vi "Format Technique (Depreciated).vi"(8 "error in (no error)":errorcluster, 9 "Technique in":T1, 10 "Technique Parameters in":variant, 11 "Potentiostat Galvanostat in":refnum<class "Potentiostat Galvanostat.lvclass">) -> (0 "error out":errorcluster, 1 "Technique Parameters out":T2 {"Parameter Type" items=["I32 (Long)", "BOOL (Boolean)", "SGL (Single Precision)"]}, 3 "Potentiostat Galvanostat out":refnum<class "Potentiostat Galvanostat.lvclass">)   [LabVIEW 2018, in "Potentiostat Galvanostat.lvclass"]
uses:
  Potentiostat Galvanostat.lvclass
  Controls/Technique Parameters.ctl
  Controls/Technique Parameter.ctl
  Controls/Parameter Type.ctl
  Controls/Technique List.ctl
  Controls/CA Parameters.ctl
  Controls/CA Internal Parameters.ctl
  Controls/CP Internal Parameters.ctl
  Controls/CP Parameters.ctl
  Controls/OCV Internal Parameters.ctl
  Controls/OCV Parameters.ctl
  Controls/CV Internal Parameters.ctl
  Controls/CV Parameters.ctl
  Controls/PEIS Internal Parameters.ctl
  Controls/PEIS Parameters.ctl
  Controls/GEIS Internal Parameters.ctl
  Controls/GEIS Parameters.ctl
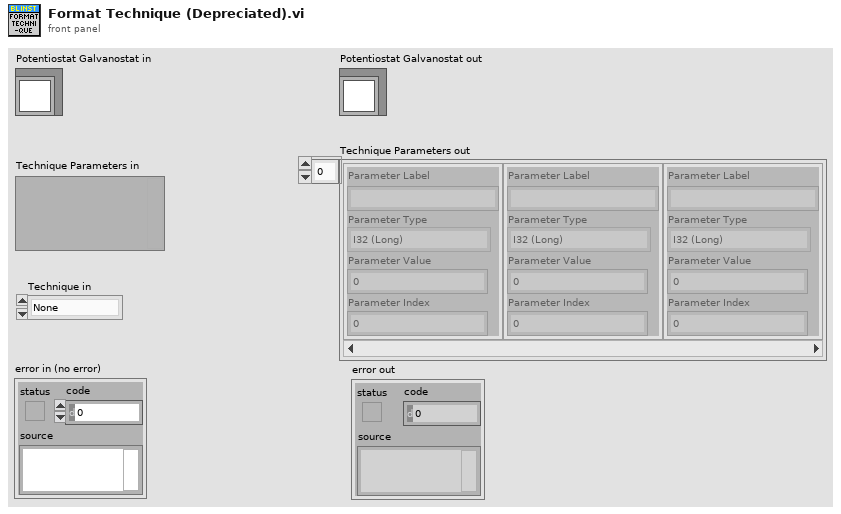
[diagram p1: front panel]
types:
  T1 = typedef "Potentiostat Galvanostat.lvclass/Technique List.ctl" = enum16{"None", "ocv", "cv", "biovscan", "ca", "cp", "iscan", "vscan", "lasv", "load", "pow", "peis", "geis", "seisp", "seisg", "dpv", "swv", "npv", "mpv", "dnpv", "dpa", "evt", "lp", "gc", "cpp", "pdp", "psp", "zra", "ircmp", "pzir", "gzir", "loop", "TO", "TI", "TOS", "vscanlimit", "iscanlimit", "mp", "casp", "casg", "calimit", "cplimit"}
  T2 = typedef "Potentiostat Galvanostat.lvclass/Technique Parameters.ctl" = T3[]
  T3 = typedef "Potentiostat Galvanostat.lvclass/Technique Parameter.ctl" = cluster{"Parameter Label":string, "Parameter Type":T4, "Parameter Value":i32, "Parameter Index":i32}
  T4 = typedef "Potentiostat Galvanostat.lvclass/Parameter Type.ctl" = i32
  T5 = typedef "Potentiostat Galvanostat.lvclass/GEIS Parameters.ctl" = cluster{"Initial frequency (Hz)":sgl, "sweep linear/logarithmic":bool, "Number of frequencies":i32, "Final frequency (Hz)":sgl, "Sine amplitude (A)":sgl, "No. of repeat times":i32, "No. of period to wait\nbefore each frequency":sgl, "Non-stationary correction":bool, "I Range":u16, "Bandwidth":u16, "CE to ground Mode":u16, "Step duration (s)":sgl, "Record every dE (V)":sgl, "Record every dt (s)":sgl, "Initial current step (A)":sgl, "Current step vs initial one":bool}
  T6 = typedef "Potentiostat Galvanostat.lvclass/GEIS Internal Parameters.ctl" = cluster{"Step_number":i32, "Initial_Current_step":sgl, "vs_initial ":bool, "Final_Current_step":sgl, "vs_final":bool, "Duration_step":sgl, "Record_every_dE":sgl, "Record_every_dT":sgl, "Initial_frequency":sgl, "sweep":bool, "Final_frequency":sgl, "Frequency_number":i32, "Amplitude_Current":sgl, "Wait_for_steady":sgl, "Average_N_times":i32, "Correction":bool, "I_Range":u16, "Bandwidth":u16, "em":u16, "ce":u16}
  T7 = typedef "Potentiostat Galvanostat.lvclass/PEIS Parameters.ctl" = cluster{"Step duration (s)":sgl, "Record every dI (A)":sgl, "Record every dt (s)":sgl, "Initial voltage step (V)":sgl, "Voltage step vs initial one":bool, "Initial frequency (Hz)":sgl, "sweep linear/logarithmic":bool, "Number of frequencies":i32, "Final frequency (Hz)":sgl, "Sine amplitude (V)":sgl, "No. of repeat times":i32, "No. of period to wait\nbefore each frequency":sgl, "Non-stationary correction":bool, "I Range":u16, "Bandwidth":u16, "CE to ground Mode":u16}
  T8 = typedef "Potentiostat Galvanostat.lvclass/PEIS Internal Parameters.ctl" = cluster{"Step_number":i32, "Initial_Voltage_step":sgl, "vs_initial":bool, "Final_Voltage_step":sgl, "vs_final":bool, "Duration_step":sgl, "Record_every_dI":sgl, "Record_every_dT":sgl, "Initial_frequency":sgl, "sweep":bool, "Final_frequency":sgl, "Frequency_number":i32, "Amplitude_Voltage":sgl, "Wait_for_steady":sgl, "Average_N_times":i32, "Correction":bool, "I_Range":u16, "Bandwidth":u16, "em":u16, "ce":u16}
  T9 = typedef "Potentiostat Galvanostat.lvclass/CV Parameters.ctl" = cluster{"Ei Params":cluster{"Current step vs initial one (Ei)":bool, "Voltage step (V) (Ei)":sgl, "slew rate array (mV/s) (Ei)":sgl}, "E1 Params":cluster{"Current step vs initial one (E1)":bool, "Voltage step (V) (E1)":sgl, "slew rate array (mV/s) (E1)":sgl}, "E2 Params":cluster{"Current step vs initial one (E2)":bool, "Voltage step (V) (E2)":sgl, "slew rate array (mV/s) (E2)":sgl}, "Ef Params":cluster{"Current step vs initial one (Ef)":bool, "Voltage step (V) (Ef)":sgl, "slew rate array (mV/s) (Ef)":sgl}, "Number of cycle":i32, "recording on dE (V)":sgl, "average every dE":bool, "Begin step accumulation (1 = 100% of step)":sgl, "End step accumulation ( 1 = 100% of step)":sgl, "I range":u16, "Bandwidth":u16, "Ewe range":u16, "CE to ground Mode":u16}
  T10 = typedef "Potentiostat Galvanostat.lvclass/CV Internal Parameters.ctl" = cluster{"Voltage_steps":cluster{"vs_initial":bool, "Voltage_step":sgl, "Scan_Rate":sgl}[], "N_Cycles":i32, "Record_every_dE":sgl, "Average_over_dE":bool, "Begin_measuring_I":sgl, "End_measuring_I":sgl, "I_Range":u16, "E_Range":u16, "Bandwidth":u16, "em":u16, "ce":u16, "Scan_number":u16, "tb":sgl}
  T11 = typedef "Potentiostat Galvanostat.lvclass/OCV Parameters.ctl" = cluster{"Rest duration (s)":sgl, "Record every dE (V)":sgl, "Record every dT (s)":sgl, "Ewe range":u16, "CE to ground Mode":u16}
  T12 = typedef "Potentiostat Galvanostat.lvclass/OCV Internal Parameters.ctl" = cluster{"Rest_time_T":sgl, "Record_every_dE":sgl, "Record_every_dT":sgl, "E_Range":u16, "em":u16, "ce":u16, "tb":sgl}
  T13 = typedef "Potentiostat Galvanostat.lvclass/CP Parameters.ctl" = cluster{"Current Steps":cluster{"Current step vs initial\none":bool, "Current step (A)":sgl, "Duration step (s)":sgl}[], "No. of steps":i32, "Record every dt (s)":sgl, "Record every dE (V)":sgl, "No. of times\ntechnique is repeated":i32, "I range":u16, "Ewe range":u16, "Bandwidth":u16, "CE to ground Mode":u16}
  T14 = typedef "Potentiostat Galvanostat.lvclass/CP Internal Parameters.ctl" = cluster{"Current_steps":cluster{"vs_initial":bool, "Current_step":sgl, "Duration_step":sgl}[], "Step_number":i32, "N_Cycles":i32, "Record_every_dE":sgl, "Record_every_dT":sgl, "I_Range":u16, "E_Range":u16, "Bandwidth":u16, "em":u16, "ce":u16, "tb":sgl}
  T15 = typedef "Potentiostat Galvanostat.lvclass/CA Internal Parameters.ctl" = cluster{"tb":sgl, "Voltage_steps":cluster{"vs_initial":bool, "Voltage_step":sgl, "Duration_step":sgl}[], "Step_number":i32, "N_Cycles":i32, "Record_every_dI":sgl, "Record_every_dT":sgl, "I_Range":u16, "E_Range":u16, "Bandwidth":u16, "em":u16, "ce":u16}
  T16 = typedef "Potentiostat Galvanostat.lvclass/CA Parameters.ctl" = cluster{"Voltage Steps":cluster{"Voltage step vs initial one":bool, "Voltage step (V)":sgl, "Duration step (s)":sgl}[], "No. of steps":i32, "Record every dt (s)":sgl, "Record every dI (A)":sgl, "No. of times\ntechnique is repeated":i32, "I range":u16, "Ewe range":u16, "Bandwidth":u16, "CE to ground Mode":u16}
  T17 = cluster{"Voltage step vs initial one":bool, "Voltage step (V)":sgl, "Duration step (s)":sgl}[]
  T18 = cluster{"Current step vs initial\none":bool, "Current step (A)":sgl, "Duration step (s)":sgl}[]
  T19 = cluster{"Current step vs initial one (Ei)":bool, "Voltage step (V) (Ei)":sgl, "slew rate array (mV/s) (Ei)":sgl}
  T20 = cluster{"Current step vs initial one (E1)":bool, "Voltage step (V) (E1)":sgl, "slew rate array (mV/s) (E1)":sgl}
  T21 = cluster{"Current step vs initial one (E2)":bool, "Voltage step (V) (E2)":sgl, "slew rate array (mV/s) (E2)":sgl}
  T22 = cluster{"Current step vs initial one (Ef)":bool, "Voltage step (V) (Ef)":sgl, "slew rate array (mV/s) (Ef)":sgl}
  T23 = cluster{"Current step vs initial one (Ef)":bool, "Voltage step (V) (Ef)":sgl, "slew rate array (mV/s) (Ef)":sgl}[]
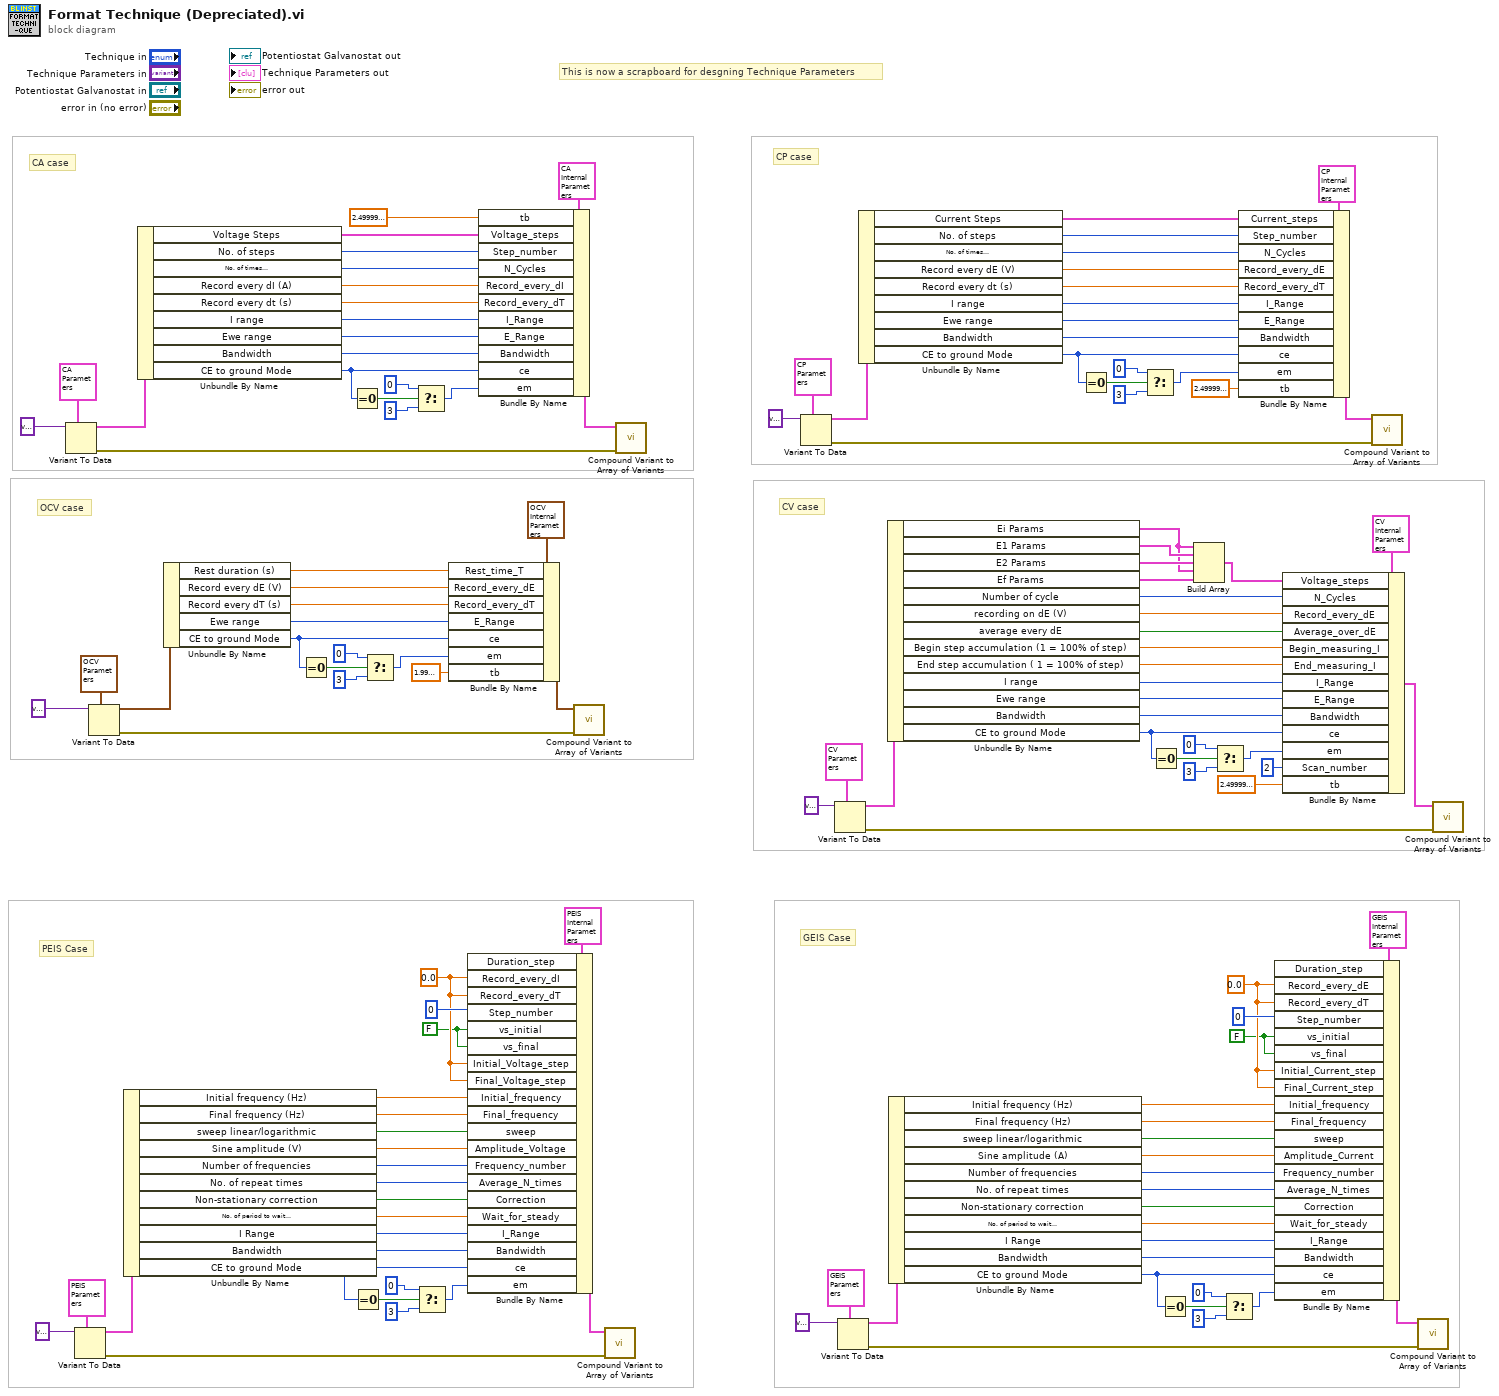
[diagram p0: block diagram]
diagram:
  w18 = FALSE ("vs_initial")
  w19 = sgl 0.0 ("Duration_step")
  w26 = FALSE ("vs_initial")
  w27 = sgl 0.0 ("Duration_step")
  # "This is now a scrapboard for desgning Technique Parameters"
  # "GEIS Case"
  # "PEIS Case"
  # "CV case"
  # "OCV case"
  # "CP case"
  # "CA case"
  n1 = Variant To Data(type=T16 {"Voltage Steps"=[{"Voltage step vs initial one"=TRUE, "Voltage step (V)"=0.0, "Duration step (s)"=1.0}, {"Voltage step vs initial one"=TRUE, "Voltage step (V)"=0.1, "Duration step (s)"=1.0}, {"Voltage step vs initial one"=TRUE, "Voltage step (V)"=0.2, "Duration step (s)"=1.0}], "No. of steps"=2, "Record every dt (s)"=0.01, "Record every dI (A)"=1e-05, "No. of times\ntechnique is repeated"=0, "I range"=12, "Ewe range"=3, "Bandwidth"=5, "CE to ground Mode"=0} ("CA Parameters"), Variant=variant ("Technique Parameters in")) -> (data=w114:T16, error out=w111:errorcluster)  [unwired: 1 in]
  n2 = Variant To Data(type=T7 {"Step duration (s)"=1.0, "Record every dI (A)"=0.1, "Record every dt (s)"=0.1, "Initial voltage step (V)"=0.0, "Voltage step vs initial one"=TRUE, "Initial frequency (Hz)"=0.0, "sweep linear/logarithmic"=TRUE, "Number of frequencies"=51, "Final frequency (Hz)"=1.0, "Sine amplitude (V)"=0.01, "No. of repeat times"=1, "No. of period to wait\nbefore each frequency"=2.0, "Non-stationary correction"=TRUE, "I Range"=12, "Bandwidth"=5, "CE to ground Mode"=0} ("PEIS Parameters"), Variant=variant ("Technique Parameters in")) -> (data=w25:T7, error out=w30:errorcluster)  [unwired: 1 in]
  n3 = Variant To Data(type=T11 {"Rest duration (s)"=1.0, "Record every dE (V)"=0.01, "Record every dT (s)"=0.01, "Ewe range"=3, "CE to ground Mode"=0} ("OCV Parameters"), Variant=variant ("Technique Parameters in")) -> (data=w79:T11, error out=w76:errorcluster)  [unwired: 1 in]
  n4 = Unbundle By Name(w25) -> ("Initial frequency (Hz)"=w48:sgl, "Final frequency (Hz)"=w47:sgl, "sweep linear/logarithmic"=w46:bool, "Sine amplitude (V)"=w45:sgl, "Number of frequencies"=w44:i32, "No. of repeat times"=w43:i32, "Non-stationary correction"=w42:bool, "No. of period to wait\nbefore each frequency"=w41:sgl, "I Range"=w40:u16, "Bandwidth"=w39:u16, "CE to ground Mode"=w33:u16)
  n5 = Unbundle By Name(w114) -> ("Voltage Steps"=w127:T17, "No. of steps"=w128:i32, "No. of times\ntechnique is repeated"=w126:i32, "Record every dI (A)"=w125:sgl, "Record every dt (s)"=w124:sgl, "I range"=w121:u16, "Ewe range"=w122:u16, "Bandwidth"=w123:u16, "CE to ground Mode"=w116:u16)
  n6 = Unbundle By Name(w79) -> ("Rest duration (s)"=w89:sgl, "Record every dE (V)"=w88:sgl, "Record every dT (s)"=w87:sgl, "Ewe range"=w86:u16, "CE to ground Mode"=w81:u16)
  n7 = Equal To 0?(x=w81) -> (x = 0?=w84:bool)
  n8 = Equal To 0?(x=w116) -> (x = 0?=w119:bool)
  n9 = Equal To 0?(x=w33) -> (x = 0?=w36:bool)
  n10 = Select(t=u16 0, s=w84, f=u16 3) -> (s? t:f=w80:u16)
  n11 = Select(t=u16 0, s=w119, f=u16 3) -> (s? t:f=w115:u16)
  n12 = Select(t=u16 0, s=w36, f=u16 3) -> (s? t:f=w32:u16)
  n13 = Bundle By Name(cluster=T12 {"Rest_time_T"=1.0, "Record_every_dE"=0.01, "Record_every_dT"=0.01, "E_Range"=3, "em"=1, "ce"=0, "tb"=2e-05} ("OCV Parameters"), "Rest_time_T"=w89, "Record_every_dE"=w88, "Record_every_dT"=w87, "E_Range"=w86, "ce"=w81, "em"=w80, "tb"=sgl 2e-05) -> (w75:T12)
  n14 = Bundle By Name(cluster=T8 {"Step_number"=0, "Initial_Voltage_step"=0.0, "vs_initial"=TRUE, "Final_Voltage_step"=1.0, "vs_final"=FALSE, "Duration_step"=1.0, "Record_every_dI"=0.1, "Record_every_dT"=0.1, "Initial_frequency"=100000.0, "sweep"=FALSE, "Final_frequency"=1.0, "Frequency_number"=51, "Amplitude_Voltage"=0.01, "Wait_for_steady"=2.0, "Average_N_times"=1, "Correction"=TRUE, "I_Range"=12, "Bandwidth"=5, "em"=1, "ce"=0} ("PEIS Parameters"), "Duration_step"=w27, "Record_every_dI"=w27, "Record_every_dT"=w27, "Step_number"=0, "vs_initial"=w26, "vs_final"=w26, "Initial_Voltage_step"=w27, "Final_Voltage_step"=w27, "Initial_frequency"=w48, "Final_frequency"=w47, "sweep"=w46, "Amplitude_Voltage"=w45, "Frequency_number"=w44, "Average_N_times"=w43, "Correction"=w42, "Wait_for_steady"=w41, "I_Range"=w40, "Bandwidth"=w39, "ce"=w33, "em"=w32) -> (w31:T8)
  n15 = Bundle By Name(cluster=T15 {"tb"=2.5e-05, "Voltage_steps"=[{"vs_initial"=TRUE, "Voltage_step"=0.0, "Duration_step"=1.0}, {"vs_initial"=TRUE, "Voltage_step"=0.1, "Duration_step"=1.0}, {"vs_initial"=TRUE, "Voltage_step"=0.2, "Duration_step"=1.0}], "Step_number"=2, "N_Cycles"=0, "Record_every_dI"=1e-05, "Record_every_dT"=0.01, "I_Range"=8, "E_Range"=3, "Bandwidth"=5, "em"=1, "ce"=0} ("CA Internal Parameters"), "tb"=sgl 2.5e-05, "Voltage_steps"=w127, "Step_number"=w128, "N_Cycles"=w126, "Record_every_dI"=w125, "Record_every_dT"=w124, "I_Range"=w121, "E_Range"=w122, "Bandwidth"=w123, "ce"=w116, "em"=w115) -> (w112:T15)
  n16 = call "Compound Variant to Array of Variants.vi"("error in (no error)"=w76, "Array/Cluster Variant"=w75) -> ()  [unwired: 8 in, 2 out]
  n17 = call "Compound Variant to Array of Variants.vi"("error in (no error)"=w30, "Array/Cluster Variant"=w31) -> ()  [unwired: 8 in, 2 out]
  n18 = call "Compound Variant to Array of Variants.vi"("error in (no error)"=w111, "Array/Cluster Variant"=w112) -> ()  [unwired: 8 in, 2 out]
  n19 = Variant To Data(type=T13 {"Current Steps"=[{"Current step vs initial\none"=FALSE, "Current step (A)"=0.0, "Duration step (s)"=1.0}, {"Current step vs initial\none"=FALSE, "Current step (A)"=0.001, "Duration step (s)"=1.0}, {"Current step vs initial\none"=FALSE, "Current step (A)"=0.005, "Duration step (s)"=1.0}], "No. of steps"=2, "Record every dt (s)"=0.05, "Record every dE (V)"=0.005, "No. of times\ntechnique is repeated"=0, "I range"=8, "Ewe range"=3, "Bandwidth"=5, "CE to ground Mode"=0} ("CP Parameters"), Variant=variant ("Technique Parameters in")) -> (data=w93:T13, error out=w94:errorcluster)  [unwired: 1 in]
  n20 = Variant To Data(type=T9 {"Ei Params"={"Current step vs initial one (Ei)"=TRUE, "Voltage step (V) (Ei)"=0.0, "slew rate array (mV/s) (Ei)"=0.1}, "E1 Params"={"Current step vs initial one (E1)"=FALSE, "Voltage step (V) (E1)"=0.1, "slew rate array (mV/s) (E1)"=0.1}, "E2 Params"={"Current step vs initial one (E2)"=FALSE, "Voltage step (V) (E2)"=-0.2, "slew rate array (mV/s) (E2)"=0.1}, "Ef Params"={"Current step vs initial one (Ef)"=TRUE, "Voltage step (V) (Ef)"=0.0, "slew rate array (mV/s) (Ef)"=0.1}, "Number of cycle"=1, "recording on dE (V)"=0.01, "average every dE"=TRUE, "Begin step accumulation (1 = 100% of step)"=0.5, "End step accumulation ( 1 = 100% of step)"=0.75, "I range"=12, "Bandwidth"=5, "Ewe range"=3, "CE to ground Mode"=0} ("CV Parameters"), Variant=variant ("Technique Parameters in")) -> (data=w49:T9, error out=w53:errorcluster)  [unwired: 1 in]
  n21 = Variant To Data(type=T5 {"Initial frequency (Hz)"=100000.0, "sweep linear/logarithmic"=FALSE, "Number of frequencies"=51, "Final frequency (Hz)"=1.0, "Sine amplitude (A)"=0.001, "No. of repeat times"=1, "No. of period to wait\nbefore each frequency"=2.0, "Non-stationary correction"=TRUE, "I Range"=12, "Bandwidth"=5, "CE to ground Mode"=0, "Step duration (s)"=1.0, "Record every dE (V)"=0.1, "Record every dt (s)"=0.1, "Initial current step (A)"=0.0, "Current step vs initial one"=TRUE} ("GEIS Parameters"), Variant=variant ("Technique Parameters in")) -> (data=w3:T5, error out=w5:errorcluster)  [unwired: 1 in]
  n22 = Unbundle By Name(w93) -> ("Current Steps"=w110:T18, "No. of steps"=w109:i32, "No. of times\ntechnique is repeated"=w108:i32, "Record every dE (V)"=w106:sgl, "Record every dt (s)"=w107:sgl, "I range"=w105:u16, "Ewe range"=w104:u16, "Bandwidth"=w103:u16, "CE to ground Mode"=w97:u16)
  n23 = Unbundle By Name(w49) -> ("Ei Params"=w57:T19, "E1 Params"=w59:T20, "E2 Params"=w58:T21, "Ef Params"=w56:T22, "Number of cycle"=w73:i32, "recording on dE (V)"=w72:sgl, "average every dE"=w71:bool, "Begin step accumulation (1 = 100% of step)"=w70:sgl, "End step accumulation ( 1 = 100% of step)"=w69:sgl, "I range"=w68:u16, "Ewe range"=w67:u16, "Bandwidth"=w66:u16, "CE to ground Mode"=w62:u16)
  n24 = Unbundle By Name(w3) -> ("Initial frequency (Hz)"=w17:sgl, "Final frequency (Hz)"=w16:sgl, "sweep linear/logarithmic"=w15:bool, "Sine amplitude (A)"=w14:sgl, "Number of frequencies"=w13:i32, "No. of repeat times"=w12:i32, "Non-stationary correction"=w11:bool, "No. of period to wait\nbefore each frequency"=w10:sgl, "I Range"=w9:u16, "Bandwidth"=w8:u16, "CE to ground Mode"=w7:u16)
  n25 = Equal To 0?(x=w97) -> (x = 0?=w100:bool)
  n26 = Select(t=u16 0, s=w100, f=u16 3) -> (s? t:f=w96:u16)
  n27 = Equal To 0?(x=w62) -> (x = 0?=w65:bool)
  n28 = Equal To 0?(x=w7) -> (x = 0?=w23:bool)
  n29 = Build Array(w57, w59, w58, w57, w56) -> (w55:T23)
  n30 = Select(t=u16 0, s=w65, f=u16 3) -> (s? t:f=w61:u16)
  n31 = Select(t=u16 0, s=w23, f=u16 3) -> (s? t:f=w20:u16)
  n32 = Bundle By Name(cluster=T14 {"Current_steps"=[{"vs_initial"=FALSE, "Current_step"=0.0, "Duration_step"=1.0}, {"vs_initial"=FALSE, "Current_step"=0.001, "Duration_step"=1.0}, {"vs_initial"=FALSE, "Current_step"=0.005, "Duration_step"=1.0}], "Step_number"=2, "N_Cycles"=0, "Record_every_dE"=0.005, "Record_every_dT"=0.05, "I_Range"=8, "E_Range"=3, "Bandwidth"=5, "em"=1, "ce"=0, "tb"=2.5e-05} ("CP Parameters"), "Current_steps"=w110, "Step_number"=w109, "N_Cycles"=w108, "Record_every_dE"=w106, "Record_every_dT"=w107, "I_Range"=w105, "E_Range"=w104, "Bandwidth"=w103, "ce"=w97, "em"=w96, "tb"=sgl 2.5e-05) -> (w92:T14)
  n33 = Bundle By Name(cluster=T6 {"Step_number"=0, "Initial_Current_step"=0.0, "vs_initial "=TRUE, "Final_Current_step"=0.001, "vs_final"=TRUE, "Duration_step"=1.0, "Record_every_dE"=0.1, "Record_every_dT"=0.1, "Initial_frequency"=100000.0, "sweep"=FALSE, "Final_frequency"=1.0, "Frequency_number"=51, "Amplitude_Current"=0.001, "Wait_for_steady"=2.0, "Average_N_times"=1, "Correction"=TRUE, "I_Range"=7, "Bandwidth"=5, "em"=1, "ce"=0} ("GEIS Parameters"), "Duration_step"=w19, "Record_every_dE"=w19, "Record_every_dT"=w19, "Step_number"=0, "vs_initial"=w18, "vs_final"=w18, "Initial_Current_step"=w19, "Final_Current_step"=w19, "Initial_frequency"=w17, "Final_frequency"=w16, "sweep"=w15, "Amplitude_Current"=w14, "Frequency_number"=w13, "Average_N_times"=w12, "Correction"=w11, "Wait_for_steady"=w10, "I_Range"=w9, "Bandwidth"=w8, "ce"=w7, "em"=w20) -> (w4:T6)
  n34 = Bundle By Name(cluster=T10 {"Voltage_steps"=[], "N_Cycles"=1, "Record_every_dE"=0.01, "Average_over_dE"=TRUE, "Begin_measuring_I"=0.5, "End_measuring_I"=0.75, "I_Range"=12, "E_Range"=3, "Bandwidth"=5, "em"=1, "ce"=0, "Scan_number"=2, "tb"=2.5e-05} ("CV Parameters"), "Voltage_steps"=w55, "N_Cycles"=w73, "Record_every_dE"=w72, "Average_over_dE"=w71, "Begin_measuring_I"=w70, "End_measuring_I"=w69, "I_Range"=w68, "E_Range"=w67, "Bandwidth"=w66, "ce"=w62, "em"=w61, "Scan_number"=u16 2, "tb"=sgl 2.5e-05) -> (w51:T10)
  n35 = call "Compound Variant to Array of Variants.vi"("error in (no error)"=w94, "Array/Cluster Variant"=w92) -> ()  [unwired: 8 in, 2 out]
  n36 = call "Compound Variant to Array of Variants.vi"("error in (no error)"=w5, "Array/Cluster Variant"=w4) -> ()  [unwired: 8 in, 2 out]
  n37 = call "Compound Variant to Array of Variants.vi"("error in (no error)"=w53, "Array/Cluster Variant"=w51) -> ()  [unwired: 8 in, 2 out]
